vi "ICNC Write Position.vi"(5 "PositionB":i32, 6 "PositionA":i32, 7 "PositionZ":i32, 8 "error in (no error)":errorcluster caption="entrée d'erreur (pas d'erreur)", 9 "PositionY":i32, 10 "PositionX":i32, 11 "Axis":u32) -> (0 "error out":errorcluster caption="sortie d'erreur", 3 "function return":u32)   [LabVIEW 2017, in "ICNC2.lvlib"]
doc: "DWORD ICNC_WritePosition( DWORD Axis,\n INT PositionX=0,\n INT PositionY=0,\n INT PositionZ=0,\n INT PositionA=0,\n INT PositionB=0);"
uses:
  ICNC2.lvlib
  <userlib>/ICNC/ICNC2.dll
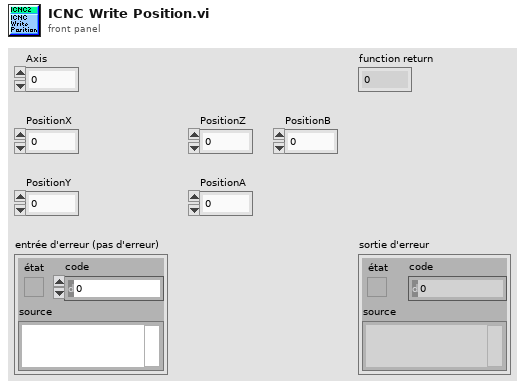
[diagram p1: front panel]
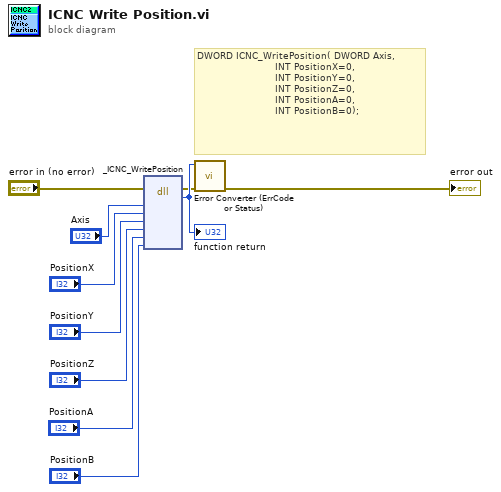
[diagram p0: block diagram]
diagram:
  # "DWORD ICNC_WritePosition( DWORD Axis,\n                          INT PositionX=0,\n                          INT PositionY=0,\n                          INT PositionZ=0,\n                          INT PositionA=0,\n                          INT PositionB=0);"
  n1 = dll-call lib="C:/Program Files (x86)/National Instruments/LabVIEW 2017/user.lib/ICNC/ICNC2.*" fn="_ICNC_WritePosition"(error in="error in (no error)", "Axis"="Axis", "PositionX"="PositionX", "PositionY"="PositionY", "PositionZ"="PositionZ", "PositionA"="PositionA", "PositionB"="PositionB") -> (error out=w2:errorcluster, w10:u32)  [unwired: 8 in, 1 out]
  "function return" <- w10
  n2 = call "Error Converter (ErrCode or Status).vi"("error in (no error)"=w2, "error code"=w10) -> ("error out"=→"error out":errorcluster)  [unwired: 9 in]
